vi "Do_SetApplicationConfiguration.vi"(8 "Error In":errorcluster, 9 "StartupConfiguration":string, 10 "ConfigSource":refnum<class "IApplicationConfiguration.lvclass">, 11 "ApplicationIn":refnum<class "Application.lvclass">) -> (0 "Error Out":errorcluster, 2 "ConfigSourceOut":refnum<class "IApplicationConfiguration.lvclass">, 3 "ApplicationOut":refnum<class "Application.lvclass">)   [LabVIEW 2021, in "Application.lvclass"]
uses:
  Application.lvclass
  Interface_TAF_IApplicationConfiguration/IApplicationConfiguration/IApplicationConfiguration.lvclass
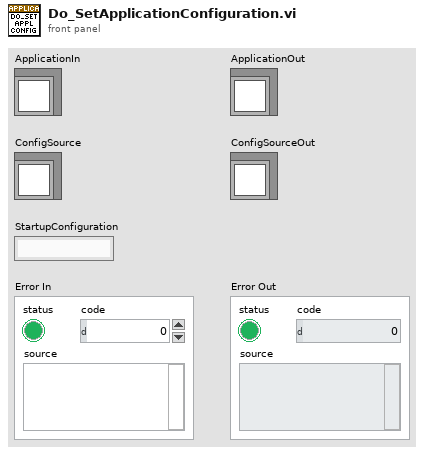
[diagram p1: front panel]
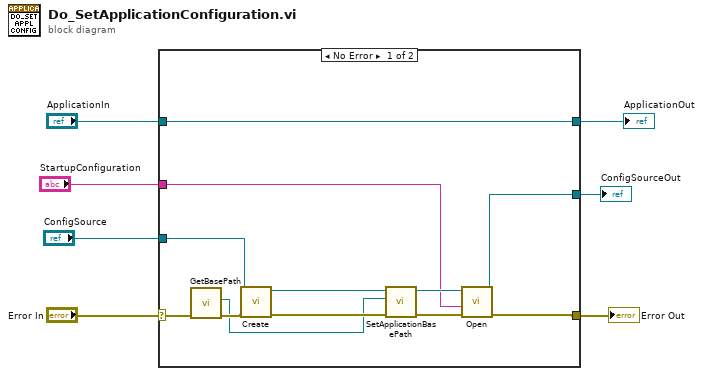
[diagram p0: block diagram]
diagram:
  n1 = case shown="No Error" "Error In" {
    selector: "Error In" -> [w15 w22]
    tunnel: [w10 w22] -> w6
    tunnel: "ConfigSource" -> [w18 w20]
    tunnel: [w19 w21] -> w3
    tunnel: "ApplicationIn" -> [w19 w21]
    tunnel: [w9 w20] -> w2
    tunnel: "StartupConfiguration" -> [w8 _]
    frame No Error {
      n2 = call "GetBasePath.vi"("Error In"=w15) -> ("Error Out"=w14:errorcluster, "BasePath"=w13:path)  [unwired: 9 in]
      n3 = call-dynamic "Create.vi"("Error In"=w14, "reference in"=w18) -> ("Error Out"=w16:errorcluster, "reference out"=w17:refnum<class "IApplicationConfiguration.lvclass">)  [unwired: 8 in]
      n4 = call-dynamic "SetApplicationBasePath.vi"("error in (no error)"=w16, "ApplicationBasePath"=w13, "reference in"=w17) -> ("error out"=w11:errorcluster, "reference out"=w12:refnum<class "IApplicationConfiguration.lvclass">)  [unwired: 7 in]
      n5 = call-dynamic "Open.vi"("Error In"=w11, "StartupConfiguration"=w8, "reference in"=w12) -> ("Error Out"=w10:errorcluster, "reference out"=w9:refnum<class "IApplicationConfiguration.lvclass">)  [unwired: 7 in]
    }
    frame Error {
    }
  }
  "Error Out" <- w6
  "ApplicationOut" <- w3
  "ConfigSourceOut" <- w2
